vi "importKeyFromStr.vi"(0 "HGF_GPG in":refnum<class "HGF_GPG.lvclass">, 1 "options file":path, 2 "keyringfile":path, 3 "Sec keyringfile":path, 4 "key":string, 5 "error in (no error)":errorcluster, 8 "Trust DB":path) -> (10 "dup Trust DB":path, 11 "success":bool, 14 "HGF_GPG out":refnum<class "HGF_GPG.lvclass">, 15 "dup options file":path, 16 "dup keyringfile":path, 17 "dup keyringfile 2":path, 19 "error out":errorcluster)   [LabVIEW 2012, in "HGF_GPG.lvlib" / "HGF_GPG.lvclass"]
doc: "Import a key from string."
uses:
  HGF_GPG.lvclass
panel:
  out "standard error":string
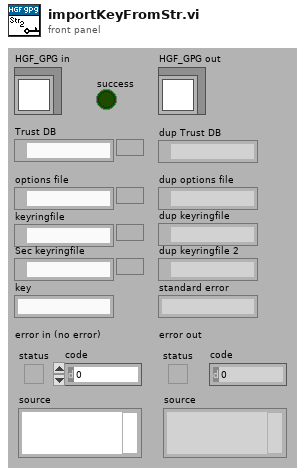
[diagram p1: front panel]
types:
  T1 = enum16{"list keys", "export", "import", "delete"}
  T2 = enum16{"open", "replace", "create", "open or create", "replace or create", "replace or create with confirmation"}
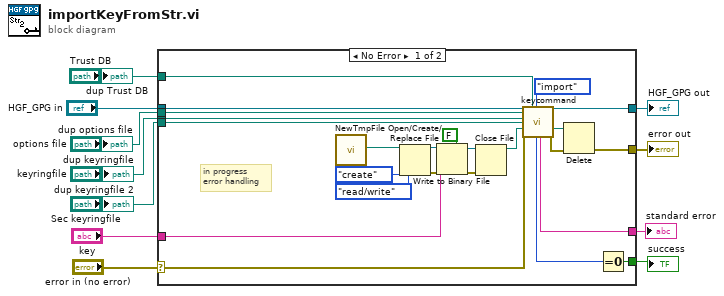
[diagram p0: block diagram]
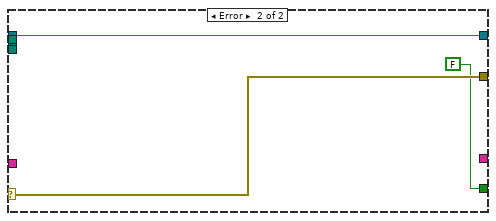
[diagram p2: hidden frame]
diagram:
  n1 = case shown="No Error" "error in (no error)" {
    selector: "error in (no error)" -> [w26 w38]
    tunnel: [w24 w38] -> w10
    tunnel: [w34 w37] -> w8
    tunnel: "HGF_GPG in" -> [w35 w37]
    tunnel: "key" -> [w29 _]
    tunnel: [w23 FALSE] -> w6
    tunnel: [w15 _] -> w5
    tunnel: "keyringfile" -> [w20 _]
    tunnel: "options file" -> [w17 _]
    tunnel: "Sec keyringfile" -> [w14 _]
    tunnel: "Trust DB" -> [w13 _]
    frame No Error {
      # "in progress\nerror handling"
      n2 = call "NewTmpFile.vi"() -> ("path"=w18:path)  [unwired: 1 in, 18 out]
      n3 = Open/Create/Replace File(file path (use dialog)=w18, operation (0:open)=T2."create", access (0:read/write)=enum16{"read/write", "read-only", "write-only"}."read/write") -> (refnum out=w30:refnum<file>, error out=w31:errorcluster)  [unwired: 1 in, 3 out]
      n4 = Write to Binary File(file (use dialog)=w30, data=w29, error in=w31, 5:FALSE ("prepend array or string size? (T)")) -> (refnum out=w27:refnum<file>, error out=w28:errorcluster)  [unwired: 3 out]
      n5 = Close File(refnum=w27, error in=w28) -> (path=w21:path)  [unwired: 1 out]
      n6 = call-dynamic "keycommand.vi"("HGF_GPG in"=w35, "options file"=w17, "keyringfile"=w20, "Sec keyringfile"=w14, "targetfile"=w21, "error in (no error)"=w26, "Trust DB"=w13, "Enum"=T1."import") -> ("return code"=w16:i32, "standard error"=w15:string, "HGF_GPG out"=w34:refnum<class "HGF_GPG.lvclass">, "dup targetfile"=w19:path, "error out"=w25:errorcluster)  [unwired: 3 in, 12 out]
      n7 = Delete(path (use dialog)=w19, error in=w25) -> (error out=w24:errorcluster)  [unwired: 5 out]
      n8 = Equal To 0?(x=w16) -> (x = 0?=w23:bool)
    }
    frame Error {
    }
  }
  "error out" <- w10
  "HGF_GPG out" <- w8
  "success" <- w6
  "standard error" <- w5
  "dup options file" <- "options file"
  "dup keyringfile" <- "keyringfile"
  "dup keyringfile 2" <- "Sec keyringfile"
  "dup Trust DB" <- "Trust DB"
